vi "PiLoN_data_processor_2D_ER.vi"(8 "PumpOffBkgd":dbl[](array[numeric]), 9 "PumpOnBkgd":dbl[](array[numeric]), 10 "Data":dbl[][](array[numeric]), 11 "# of Images":u16) -> (0 "Pump_Off":dbl[](array[numeric]), 1 "Pump_On":dbl[](array[numeric]), 2 "Raman_Gain":dbl[](array[numeric]), 3 "Raman_Gain_EX":dbl[](array[numeric]), 4 "Pump_Off2":dbl[](array[numeric]), 5 "Pump_On2":dbl[](array[numeric]), 6 "Raman_Gain2":dbl[](array[numeric]))   [LabVIEW 2015]
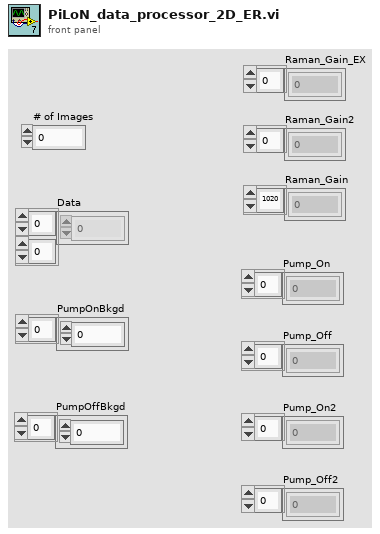
[diagram p1: front panel]
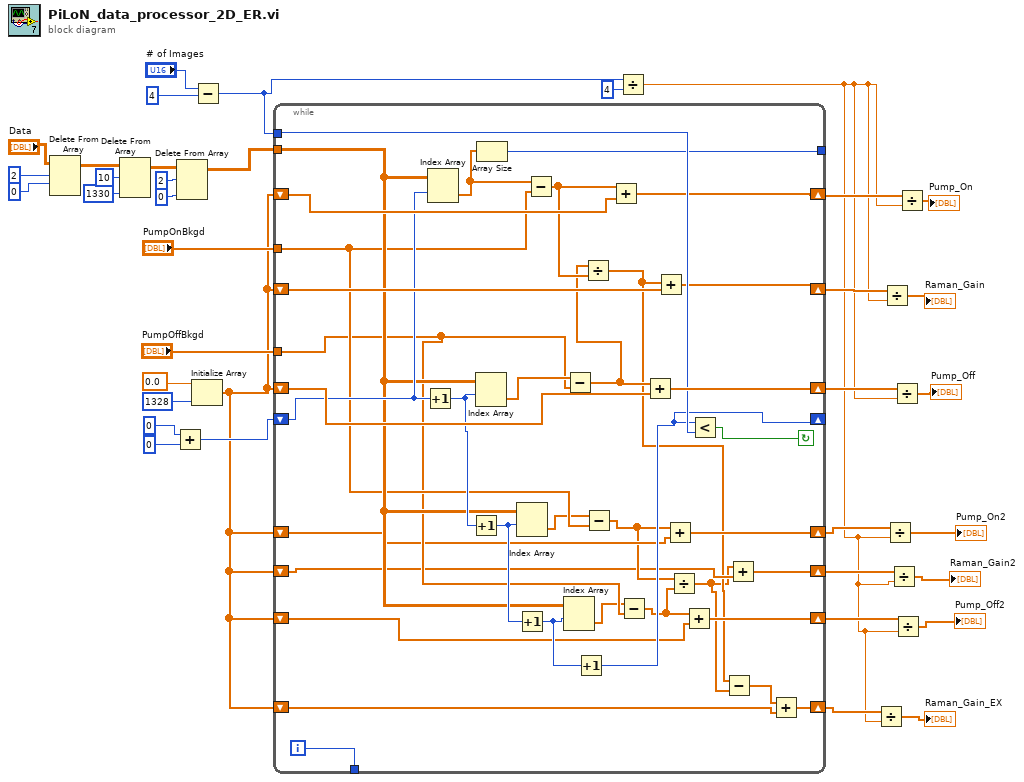
[diagram p0: block diagram]
diagram:
  n1 = Delete From Array(array="Data", length=2, index (row)=0 ("disabled index (col)")) -> (array with subset deleted=w17:dbl[][])  [unwired: 1 in, 1 out]
  n2 = Delete From Array(array=w17, length=10, index (col)=1330 ("disabled index (col)")) -> (array with subset deleted=w14:dbl[][])  [unwired: 1 in, 1 out]
  n3 = Add(x=0, y=0) -> (x+y=w26:i32)
  n4 = Delete From Array(array=w14, length=2, index (col)=0 ("disabled index (col)")) -> (array with subset deleted=w11:dbl[][])  [unwired: 1 in, 1 out]
  n5 = Initialize Array(0.0, u32 1328) -> (w4:dbl[])
  n6 = Subtract(x="# of Images", y=4) -> (x-y=w23:i32)
  n7 = while {
    tunnel: w11 -> [w56]
    shift-right: [w64] -> w22
    shift-left: w4 -> [w72]
    shift-right: [w73] -> w36
    shift-left: w4 -> [w74]
    tunnel: w23 -> [w71]
    shift-right: [w63] -> w32
    shift-left: w4 -> [w70]
    shift-right: [w68] -> _
    shift-left: w26 -> [w65]
    tunnel: "PumpOnBkgd" -> [w55]
    tunnel: "PumpOffBkgd" -> [w53]
    tunnel: [w62] -> _
    tunnel: [w59] -> _
    shift-right: [w50] -> w10
    shift-left: w4 -> [w48]
    shift-right: [w49] -> w9
    shift-left: w4 -> [w47]
    shift-right: [w43] -> w6
    shift-left: w4 -> [w44]
    shift-right: [w38] -> w3
    shift-left: w4 -> [w39]
    i -> [w59]
    stop <- w69 continue-if-true
    n8 = Increment(x=w65) -> (x+1=w58:i32)
    n9 = Index Array(array=w56, index (row)=w65) -> (element=w61:dbl[])  [unwired: 1 in]
    n10 = Increment(x=w58) -> (x+1=w57:i32)
    n11 = Index Array(array=w56, index (row)=w58) -> (element=w60:dbl[])  [unwired: 1 in]
    n12 = Array Size(array=w61) -> (size(s)=w62:i32)
    n13 = Index Array(array=w56, index (row)=w57) -> (element=w54:dbl[])  [unwired: 1 in]
    n14 = Increment(x=w57) -> (x+1=w51:i32)
    n15 = Subtract(x=w61, y=w55) -> (x-y=w67:dbl[])
    n16 = Index Array(array=w56, index (row)=w51) -> (element=w52:dbl[])  [unwired: 1 in]
    n17 = Subtract(x=w60, y=w53) -> (x-y=w66:dbl[])
    n18 = Increment(x=w51) -> (x+1=w68:i32)
    n19 = Divide(x=w66, y=w67) -> (x/y=w42:dbl[])
    n20 = Subtract(x=w54, y=w55) -> (x-y=w46:dbl[])
    n21 = Add(x=w67, y=w72) -> (x+y=w64:dbl[])
    n22 = Subtract(x=w52, y=w53) -> (x-y=w45:dbl[])
    n23 = Add(x=w66, y=w74) -> (x+y=w73:dbl[])
    n24 = Add(x=w42, y=w70) -> (x+y=w63:dbl[])
    n25 = Add(x=w46, y=w48) -> (x+y=w50:dbl[])
    n26 = Divide(x=w46, y=w45) -> (x/y=w41:dbl[])
    n27 = Add(x=w45, y=w47) -> (x+y=w49:dbl[])
    n28 = Less?(x=w68, y=w71) -> (x < y?=w69:bool)
    n29 = Subtract(x=w42, y=w41) -> (x-y=w40:dbl[])
    n30 = Add(x=w41, y=w44) -> (x+y=w43:dbl[])
    n31 = Add(x=w40, y=w39) -> (x+y=w38:dbl[])
  }
  n32 = Divide(x=w23, y=4) -> (x/y=w2:dbl)
  n33 = Divide(x=w3, y=w2) -> (x/y=→"Raman_Gain_EX":dbl[])
  n34 = Divide(x=w32, y=w2) -> (x/y=→"Raman_Gain":dbl[])
  n35 = Divide(x=w10, y=w2) -> (x/y=→"Pump_On2":dbl[])
  n36 = Divide(x=w6, y=w2) -> (x/y=→"Raman_Gain2":dbl[])
  n37 = Divide(x=w36, y=w2) -> (x/y=→"Pump_Off":dbl[])
  n38 = Divide(x=w9, y=w2) -> (x/y=→"Pump_Off2":dbl[])
  n39 = Divide(x=w22, y=w2) -> (x/y=→"Pump_On":dbl[])
